vi "PH_gentec_P-Link.set Autorange.vi"(0 "i ref in":refnum<vi>, 2 "VISA resource in":refnum<visa-resource-name>, 5 "error in":errorcluster) -> (11 "Timeout":bool, 13 "Data read":string[](array[string]), 14 "i ref out":refnum<vi>, 16 "VISA resource out":refnum<visa-resource-name>, 17 "Error":bool, 18 "Failure":bool, 19 "error out":errorcluster)   [LabVIEW 2014, in "PH_gentec_P-Link.lvlib"]
doc: "This VI writes wanted Settings to the Device and checks the result."
uses:
  PH_gentec_P-Link.lvlib
  PH_Basics/PH_Powermeter_BaseClass/PH_Powermeter_BaseClass.lvlib
  instr.lib/Gentec-P-Link/gentec-P-Link - Driver.lvlib
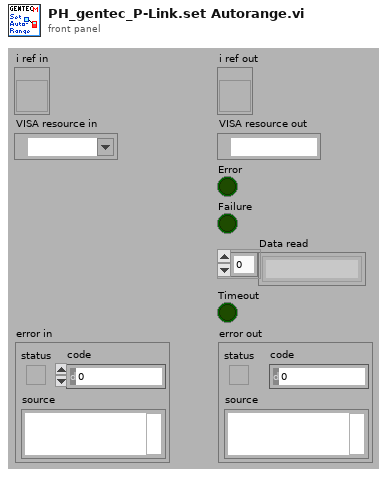
[diagram p1: front panel]
types:
  T1 = typedef "PH_gentec_P-Link.lvlib/PH_gentec_P-Link.i attribute.ctl" = cluster{"GUI References":cluster{"Wanted Head Settings":refnum<vi>, "Current Head Settings":refnum<vi>, "Set Auto Range":refnum<vi>, "Trigger Polarity":refnum<vi>, "Trigger Source":refnum<vi>, "Waveform Averages":refnum<vi>, "Continuous":refnum<vi>, "get one Value":refnum<vi>}, "Wanted Head Settings":T2, "Current Head Settings":T2}
  T2 = typedef "PH_gentec_P-Link.lvlib/PH_gentec_P-Link.Head Settings.ctl" = cluster{"Measurement Mode":T3, "Enable Anticipation":bool, "Set Auto Range":bool, "Block Signal":bool, "Set Head Attenuator":bool, "Enable SSE":bool, "Trigger Polarity":T4, "Trigger Source":T5, "Waveform Averages":T6, "Set Zero":i32, "Current Measurement":i32, "Start Data Flow":bool}
  T3 = typedef "gentec-M-Link - Driver.lvlib/gentec-M-Link.Measurement Mode.ctl" = u16
  T4 = typedef "gentec-M-Link - Driver.lvlib/gentec-M-Link.Trigger Polarity.ctl" = u16
  T5 = typedef "gentec-M-Link - Driver.lvlib/gentec-M-Link.Trigger Source.ctl" = u16
  T6 = typedef "gentec-M-Link - Driver.lvlib/gentec-M-Link.Waveform Averages.ctl" = u16
  T7 = typedef "PH_Powermeter_BaseClass.lvlib/PH_Powermeter_BaseClass.i attribute.ctl" = cluster{"GUI References":T8, "Connection":T9, "Head Attributes":T11, "VISA resource":refnum<visa-resource-name>, "Energy":T12, "Service ID Energy":i32, "Wanted Settings":T13, "Current Settings":T13}
  T8 = typedef "PH_Powermeter_BaseClass.lvlib/PH_Powermeter_BaseClass.GUI Refs.ctl" = cluster{"Head Attributes":refnum<vi>, "Energy":refnum<vi>, "Connection":refnum<vi>, "VISA Resource":refnum<vi>, "Energy evolution":refnum<vi>, "Scaling Factor":refnum<vi>, "Range":refnum<vi>, "Wavelength":refnum<vi>, "Trigger Level":refnum<vi>, "Wanted Settings":refnum<vi>, "Current Settings":refnum<vi>}
  T9 = typedef "PH_Powermeter_BaseClass.lvlib/PH_Powermeter_BaseClass.Connection.ctl" = cluster{"failed checks":i8, "Timeout":bool, "Data read":string, "Failure":bool, "Error":bool, "State":T10}
  T10 = typedef "PH_Powermeter_BaseClass.lvlib/PH_Powermeter_BaseClass.State.ctl" = enum32{"off", "operating", "opened", "checked", "connected", "Sets to change", "running"}
  T11 = typedef "PH_Powermeter_BaseClass.lvlib/PH_Powermeter_BaseClass.Head Attributes.ctl" = cluster{"Instrument Type":string, "Head Version":string, "Head Name":string, "Serial Number":string, "Firmware":string, "Sensor Type":string, "MinimumRange":u32, "Maximum Range":u32, "Min Wavelength":i32, "Max Wavelength":i32}
  T12 = typedef "PH_Powermeter_BaseClass.lvlib/PH_Powermeter_BaseClass.Energy.ctl" = cluster{"current Value":dbl, "unscaled":dbl, "Scaling Factor":dbl}
  T13 = typedef "PH_Powermeter_BaseClass.lvlib/PH_gentec_BaseClass.Head Settings.ctl" = cluster{"Trigger Level":dbl, "Wavelength":u32, "Range":u32}
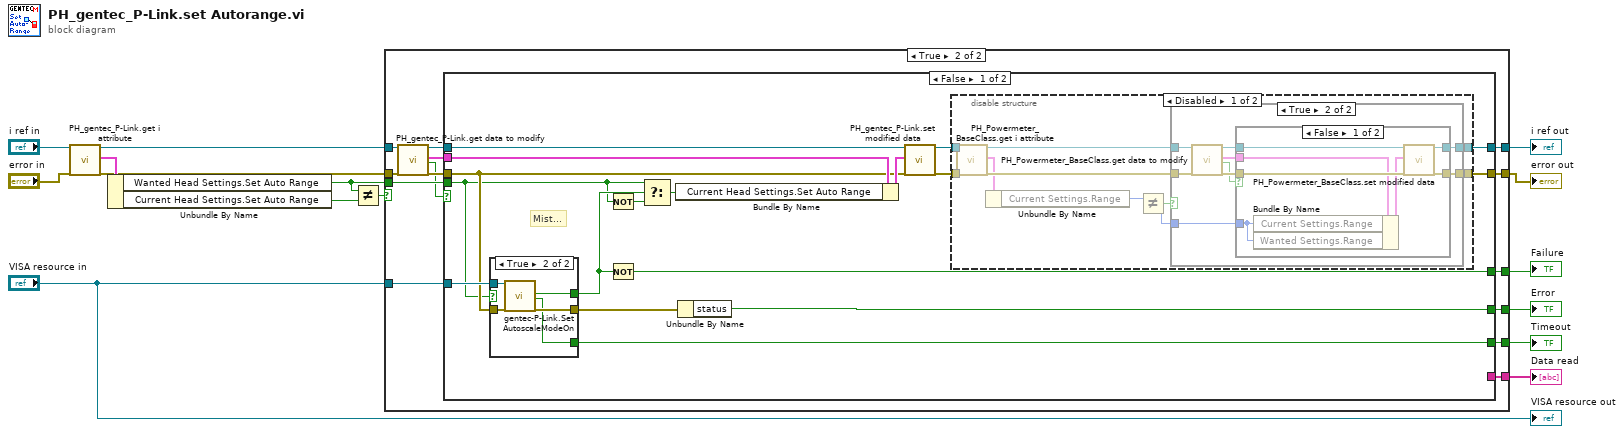
[diagram p0: block diagram]
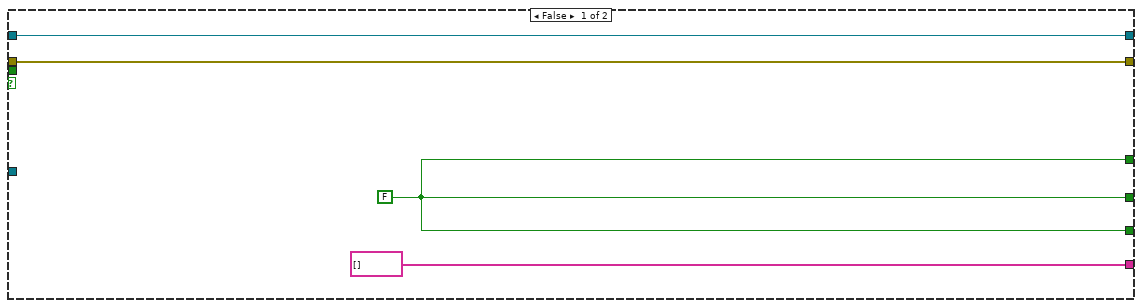
[diagram p2: hidden frame]
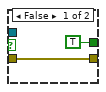
[diagram p3: hidden frame]
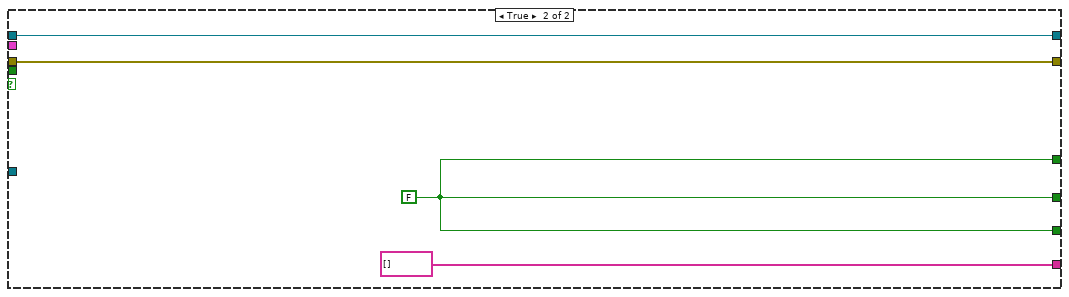
[diagram p7: hidden frame]
diagram:
  n1 = call "PH_gentec_P-Link.get i attribute.vi"("i ref in"="i ref in", "error in (no error)"="error in") -> ("i ref out"=w8:refnum<vi>, "i attribute"=w11:T1, "error out"=w10:errorcluster)  [unwired: 15 in]
  n2 = Unbundle By Name(w11) -> ("Wanted Head Settings.Set Auto Range"=w12:bool, "Current Head Settings.Set Auto Range"=w13:bool)
  n3 = Not Equal?(x=w12, y=w13) -> (x != y?=w1:bool)
  n4 = case shown="True" w1 {
    tunnel: [w18 w33] -> w15
    tunnel: [w19 w32] -> w14
    tunnel: w12 -> [_ w31]
    tunnel: w10 -> [w18 w26]
    tunnel: w8 -> [w19 w25]
    tunnel: "VISA resource in" -> [_ w24]
    tunnel: [string[] [] w23] -> w5
    tunnel: [w17 w22] -> w4
    tunnel: [w17 w21] -> w3
    tunnel: [w17 w20] -> w2
    frame False {
      w17 = FALSE
    }
    frame True {
      n5 = call "PH_gentec_P-Link.get data to modify.vi"("i ref in"=w25, "error in (no error)"=w26) -> ("i ref out"=w29:refnum<vi>, "i attribute"=w28:T1, "timed out"=w27:bool, "error out"=w30:errorcluster)  [unwired: 14 in]
      n6 = case shown="False" w27 {
        tunnel: w24 -> [w40 _]
        tunnel: [w42 w93] -> w32
        tunnel: [w41 w92] -> w33
        tunnel: w30 -> [w39 w92]
        tunnel: w29 -> [w50 w93]
        tunnel: w28 -> [w46 _]
        tunnel: w31 -> [w34 _]
        tunnel: [_ string[] []] -> w23
        tunnel: [w35 w90] -> w22
        tunnel: [w45 w90] -> w21
        tunnel: [w36 w90] -> w20
        frame False {
          # "Mist..."
          n7 = case shown="True" w34 {
            tunnel: w40 -> [_ w57]
            tunnel: w39 -> [w51 w56]
            tunnel: [w51 w55] -> w38
            tunnel: [TRUE ("Sucess?") w54] -> w37
            tunnel: [_ w53] -> w35
            frame False {
            }
            frame True {
              n8 = call "gentec-P-Link.Set AutoscaleModeOn.vi"("VISA resource name"=w57, "error in (no error)"=w56) -> ("Sucess?"=w54:bool, "TimeOut?"=w53:bool, "error out"=w55:errorcluster)  [unwired: 14 in, 1 out]
            }
          }
          n9 = Not(x=w34) -> (.not. x?=w48:bool)
          n10 = Not(x=w37) -> (.not. x?=w36:bool)
          n11 = Select(t=w34, s=w37, f=w48) -> (s? t:f=w47:bool)
          n12 = Bundle By Name(cluster=w46, "Current Head Settings.Set Auto Range"=w47) -> (w49:T1)
          n13 = Unbundle By Name(w38) -> ("status"=w45:bool)
          n14 = call "PH_gentec_P-Link.set modified data.vi"("i ref in"=w50, "i attribute"=w49, "error in (no error)"=w39) -> ("i ref out"=w44:refnum<vi>, "error out"=w43:errorcluster)  [unwired: 15 in]
          n15 = disable-structure shown="Disabled" {
            disable-tunnel: w44 -> [w62 w89]
            disable-tunnel: w43 -> [w61 w88]
            disable-tunnel: [w60 w89] -> w42
            disable-tunnel: [w59 w88] -> w41
            frame Disabled {
              n16 = call "PH_Powermeter_BaseClass.get i attribute.vi"("i ref in"=w62, "error in (no error)"=w61) -> ("i ref out"=w66:refnum<vi>, "i attribute"=w64:T7, "error out"=w65:errorcluster)  [unwired: 15 in]
              n17 = Unbundle By Name(w64) -> ("Current Settings.Range"=w63:u32)
              n18 = Not Equal?(x=w63) -> (y=w58:u32, x != y?=w67:bool)
              n19 = case shown="True" w67 {
                tunnel: [w68 w78] -> w59
                tunnel: [w69 w77] -> w60
                tunnel: w65 -> [w68 w72]
                tunnel: w66 -> [w69 w71]
                tunnel: w58 -> [_ w70]
                frame False {
                }
                frame True {
                  n20 = call "PH_Powermeter_BaseClass.get data to modify.vi"("i ref in"=w71, "error in (no error)"=w72) -> ("i ref out"=w75:refnum<vi>, "i attribute"=w74:T7, "timed out"=w73:bool, "error out"=w76:errorcluster)  [unwired: 14 in]
                  n21 = case shown="False" w73 {
                    tunnel: [w82 w87] -> w77
                    tunnel: [w81 w86] -> w78
                    tunnel: w76 -> [w84 w86]
                    tunnel: w75 -> [w85 w87]
                    tunnel: w74 -> [w83 _]
                    tunnel: w70 -> [w79 _]
                    frame False {
                      n22 = Bundle By Name(cluster=w83, "Current Settings.Range"=w79, "Wanted Settings.Range"=w79) -> (w80:T7)
                      n23 = call "PH_Powermeter_BaseClass.set modified data.vi"("i ref in"=w85, "i attribute"=w80, "error in (no error)"=w84) -> ("i ref out"=w82:refnum<vi>, "error out"=w81:errorcluster)  [unwired: 15 in]
                    }
                    frame True {
                    }
                  }
                }
              }
            }
            frame Enabled {
            }
          }
        }
        frame True {
          w90 = FALSE
        }
      }
    }
  }
  "error out" <- w15
  "i ref out" <- w14
  "Data read" <- w5
  "Timeout" <- w4
  "Error" <- w3
  "Failure" <- w2
  "VISA resource out" <- "VISA resource in"
